vi "Type Conversion.From Double (1D I32).vi"(3 "values in":dbl[](array[numeric])) -> (1 "values out":i32[](array[numeric]))   [LabVIEW 2016, in "VeriStand Data.lvlib"]
doc: "Converts the provided double float values to the specified data type, preserving the numerical value of the data."
uses:
  VeriStand Data.lvlib
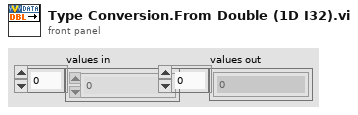
[diagram p1: front panel]
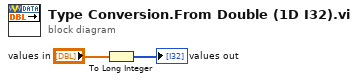
[diagram p0: block diagram]
diagram:
  n1 = To Long Integer(number="values in") -> (32bit integer=→"values out":i32[])
